vi "Event Actor.vi"(4 "Queue Nested":map{string, refnum<data-value>}(c390), 6 "Queue Self":map{string, refnum<data-value>}(c390), 8 "Queue Caller":map{string, refnum<data-value>}(c390), 9 "Queue of Event Self":refnum<queue>, 10 "Event Self Alias":string, 11 "Event Actor":refnum<class "Event Actor.lvclass">) -> ()   [LabVIEW 2021, in "jettl.lvlib" / "Base Event Actor.lvclass"]
uses:
  Base Event Actor.lvclass
  Actor/Event Actor/Event Actor.lvclass
  Msg/Msg/Msg.lvclass
  C:/git/jettl/src/jettl/Event Actor/Event Actor.lvclass
  Msg/Msgs/Event Last Ack/Event Last Ack Msg/Event Last Ack Msg.lvclass
  C:/git/jettl/src/jettl/Msg/Msg.lvclass
  jettl.lvlib
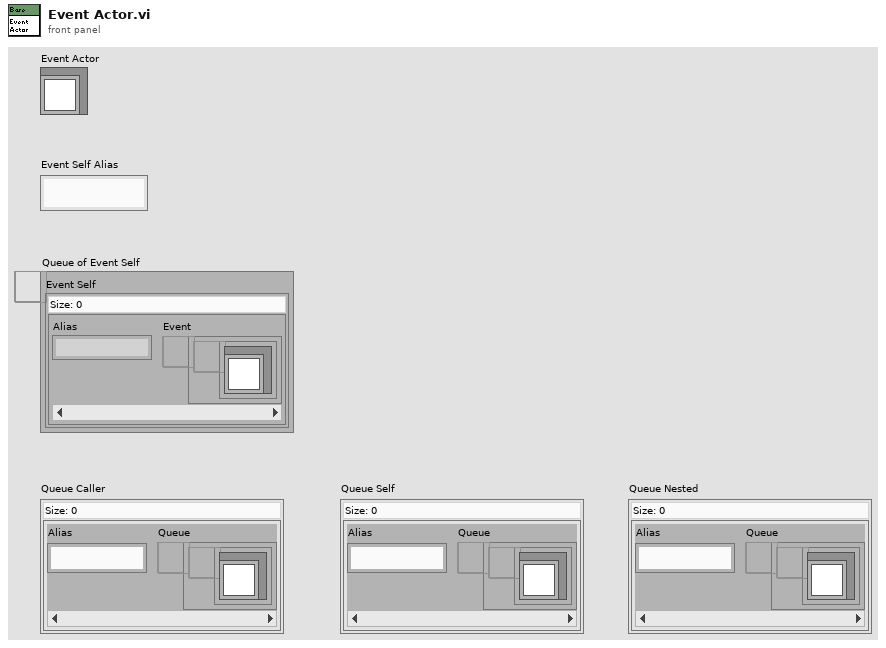
[diagram p1: front panel]
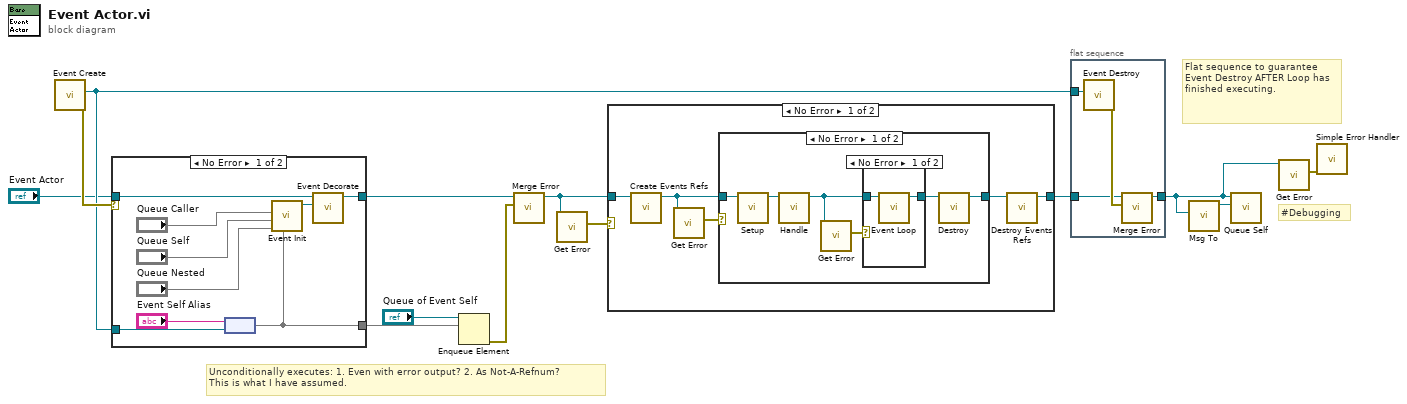
[diagram p0: block diagram]
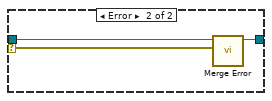
[diagram p2: hidden frame]
diagram:
  # "Flat sequence to guarantee Event Destroy AFTER Loop has finished executing."
  # "Unconditionally executes: 1. Even with error output? 2. As Not-A-Refnum?\nThis is what I have assumed."
  # "#Debugging"
  n1 = call "Event Create.vi"() -> ("error out"=w7:errorcluster, "Event"=w6:refnum<data-value>)  [unwired: 10 in]
  n2 = case shown="No Error" w7 {
    selector: w7 -> [_ w24]
    tunnel: [w14 w25] -> w11
    tunnel: "Event Actor" -> [w21 w23]
    tunnel: w6 -> [w22 _]
    tunnel: [w20 _] -> w10
    frame No Error {
      n3 = node("Event Self Alias", w22) -> (w20:map{string, refnum<data-value>})
      n4 = call "Event Init.vi"("Event Self"=w20, "Queue Nested"="Queue Nested", "Queue Self"="Queue Self", "Queue Caller"="Queue Caller") -> ("Base Event Actor out"=w15:refnum<class "Base Event Actor.lvclass">)  [unwired: 7 in]
      n5 = call-dynamic "Event Decorate.vi"("Event Actor"=w15, "Event Actor in"=w21) -> ("Event Actor out"=w14:refnum<class "Event Actor.lvclass">)  [unwired: 9 in]
    }
    frame Error {
      n6 = call-dynamic "Merge Error.vi"("Error"=w24, "Set Error in"=w23) -> ("Set Error out"=w25:refnum<class "Event Actor.lvclass">)  [unwired: 9 in]
    }
  }
  n7 = Enqueue Element(queue="Queue of Event Self", element=w10) -> (error out=w12:errorcluster)  [unwired: 2 in, 2 out]
  n8 = call-dynamic "Merge Error.vi"("Error"=w12, "Set Error in"=w11) -> ("Set Error out"=w13:refnum<class "Event Actor.lvclass">)  [unwired: 9 in]
  n9 = call-dynamic "Get Error.vi"("Actor in"=w13) -> ("Error"=w9:errorcluster)  [unwired: 10 in]
  n10 = case shown="No Error" w9 {
    tunnel: w13 -> [w30 w41]
    tunnel: [w26 w41] -> w8
    frame No Error {
      n11 = call-dynamic "Create Events Refs.vi"("Event Actor in"=w30) -> ("Event Actor out"=w28:refnum<class "Event Actor.lvclass">)  [unwired: 10 in]
      n12 = call-dynamic "Get Error.vi"("Actor in"=w28) -> ("Error"=w29:errorcluster)  [unwired: 10 in]
      n13 = case shown="No Error" w29 {
        tunnel: w28 -> [w36 w40]
        tunnel: [w31 w40] -> w27
        frame No Error {
          n14 = call-dynamic "Setup.vi"("Setup in"=w36) -> ("Setup out"=w35:refnum<class "Event Actor.lvclass">)  [unwired: 10 in]
          n15 = call-dynamic "Handle.vi"("Actor in"=w35) -> ("Actor out"=w34:refnum<class "Event Actor.lvclass">)  [unwired: 9 in, 1 out]
          n16 = call-dynamic "Get Error.vi"("Actor in"=w34) -> ("Error"=w33:errorcluster)  [unwired: 10 in]
          n17 = case shown="No Error" w33 {
            tunnel: [w37 w39] -> w32
            tunnel: w34 -> [w38 w39]
            frame No Error {
              n18 = call-dynamic "Event Loop.vi"("Event Actor in"=w38) -> ("Event Actor out"=w37:refnum<class "Event Actor.lvclass">)  [unwired: 10 in]
            }
            frame Error {
            }
          }
          n19 = call-dynamic "Destroy.vi"("Actor in"=w32) -> ("Actor out"=w31:refnum<class "Event Actor.lvclass">)  [unwired: 10 in]
        }
        frame Error {
        }
      }
      n20 = call-dynamic "Destroy Events Refs.vi"("Event Actor in"=w27) -> ("Event Actor out"=w26:refnum<class "Event Actor.lvclass">)  [unwired: 10 in]
    }
    frame Error {
    }
  }
  n21 = flat-sequence {
    tunnel: w6 -> [w44]
    tunnel: [w45] -> w1
    tunnel: w8 -> [w42]
    frame #0 {
      n22 = call "Event Destroy.vi"("Event"=w44) -> ("error out"=w43:errorcluster)  [unwired: 10 in]
      n23 = call-dynamic "Merge Error.vi"("Error"=w43, "Set Error in"=w42) -> ("Set Error out"=w45:refnum<class "Event Actor.lvclass">)  [unwired: 9 in]
    }
  }
  n24 = call "Msg To.vi"("Event Actor"=w1) -> ("Event Last Ack Msg out"=w3:refnum<class "Event Last Ack Msg.lvclass">)  [unwired: 10 in]
  n25 = call-dynamic "Queue Self.vi"("Msg"=w3, "Actor in"=w1) -> ()  [unwired: 9 in, 1 out]
  n26 = call-dynamic "Get Error.vi"("Actor in"=w1) -> ("Error"=w2:errorcluster)  [unwired: 10 in]
  n27 = call <vilib>:"Simple Error Handler.vi"("error in (no error)"=w2) -> ()  [unwired: 4 in, 5 out]
